vi "Read Startup Messages.vi"(8 "error in (no error)":errorcluster, 11 "CLI in":refnum<class "CLI.lvclass">) -> (0 "error out":errorcluster, 1 "Working Directory":path, 2 "Arguments":string[](array[string]), 3 "CLI out":refnum<class "CLI.lvclass">)   [LabVIEW 2017, in "CLI.lvclass"]
uses:
  CLI.lvclass
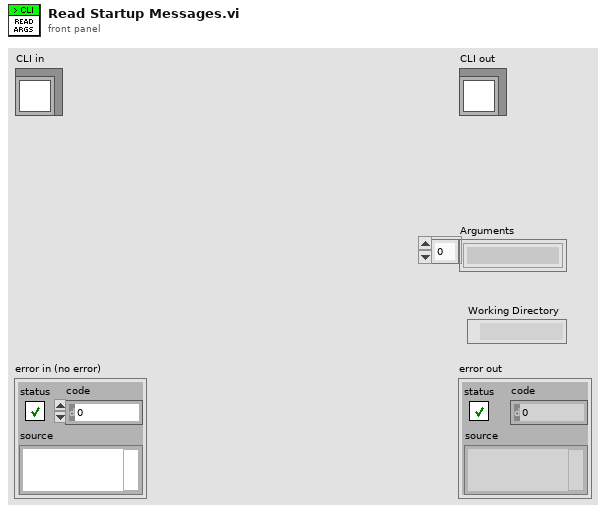
[diagram p1: front panel]
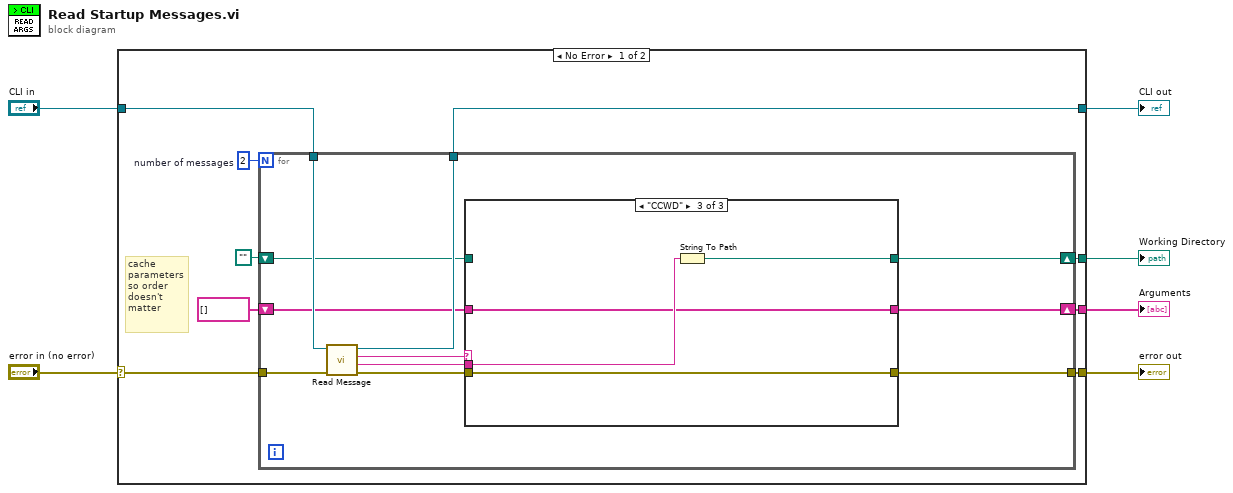
[diagram p0: block diagram]
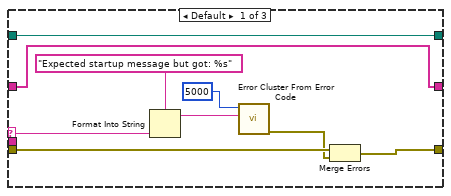
[diagram p2: hidden frame]
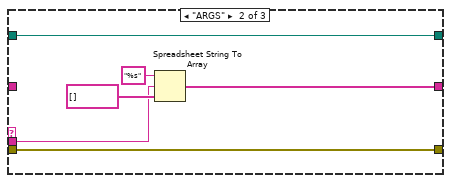
[diagram p3: hidden frame]
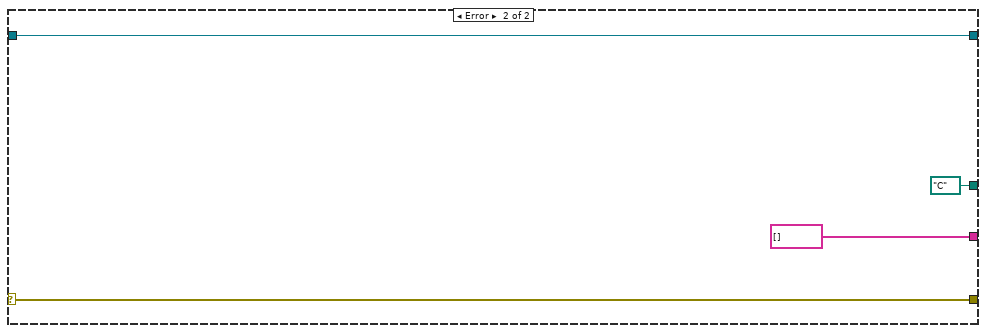
[diagram p4: hidden frame]
diagram:
  n1 = case shown="No Error" "error in (no error)" {
    selector: "error in (no error)" -> [w15 w49]
    tunnel: [w12 w49] -> w5
    tunnel: [w13 w48] -> w3
    tunnel: "CLI in" -> [w14 w48]
    tunnel: [w11 string[] []] -> w2
    tunnel: [w10 path "C:/"] -> w1
    frame No Error {
      w7 = 2  # number of messages
      # "cache\nparameters\nso order\ndoesn't\nmatter"
      n2 = for {
        N: w7 -> [_]
        tunnel: w15 -> [w26]
        tunnel: w14 -> [w25]
        tunnel: [w24] -> w13
        tunnel: [w22] -> w12
        shift-right: [w20] -> w11
        shift-left: string[] [] -> [w17]
        shift-right: [w18] -> w10
        shift-left: path "" -> [w16]
        n3 = call "Read Message.vi"("error in (no error)"=w26, "CLI in"=w25) -> ("error out"=w21:errorcluster, "Message Contents"=w19:string, "Message Type"=w23:string, "CLI out"=w24:refnum<class "CLI.lvclass">)  [unwired: 6 in]
        n4 = case shown="\"CCWD\"" w23 {
          selector: w23 -> [w31 _ _]
          tunnel: [w30 w41 w45] -> w22
          tunnel: w21 -> [w35 w41 w45]
          tunnel: [w27 w38 w42] -> w20
          tunnel: w19 -> [_ w37 w44]
          tunnel: [w28 w36 w43] -> w18
          tunnel: w17 -> [w27 _ w42]
          tunnel: w16 -> [w28 w36 _]
          frame Default {
            n5 = Format Into String(format string="Expected startup message but got: %s", w31) -> (resulting string=w32:string)  [unwired: 2 in, 1 out]
            n6 = call <vilib>:"Error Cluster From Error Code.vi"("error message (\"\")"=w32, "error code (0)"=5000) -> ("error out"=w29:errorcluster)  [unwired: 7 in]
            n7 = Merge Errors(w35, w29) -> (w30:errorcluster)
          }
          frame "ARGS" {
            n8 = Spreadsheet String To Array(format string="%s", spreadsheet string=w37, array type (2D Dbl)=string[] []) -> (array=w38:string[])  [unwired: 1 in]
          }
          frame "CCWD" {
            n9 = String To Path(string=w44) -> (path=w43:path)
          }
        }
      }
    }
    frame Error {
    }
  }
  "error out" <- w5
  "CLI out" <- w3
  "Arguments" <- w2
  "Working Directory" <- w1
